vi "Configure Watchdog.vi"(5 "Dog stop notifier":refnum<notifier>, 7 "Period":i32, 8 "error in (no error)":errorcluster, 9 "Register":u16, 10 "Modbus Handle":refnum<class "Modbus Master.lvclass">, 11 "Watchdog in":refnum<class "Watchdog.lvclass">) -> (0 "error out":errorcluster, 3 "Watchdog out":refnum<class "Watchdog.lvclass">)   [LabVIEW 2015, in "Watchdog Actor.lvlib" / "Watchdog.lvclass"]
uses:
  Watchdog.lvclass
  <vilib>/Modbus/master/Modbus Master.lvclass
  Watchdog.lvclass/Watchdog.ctl
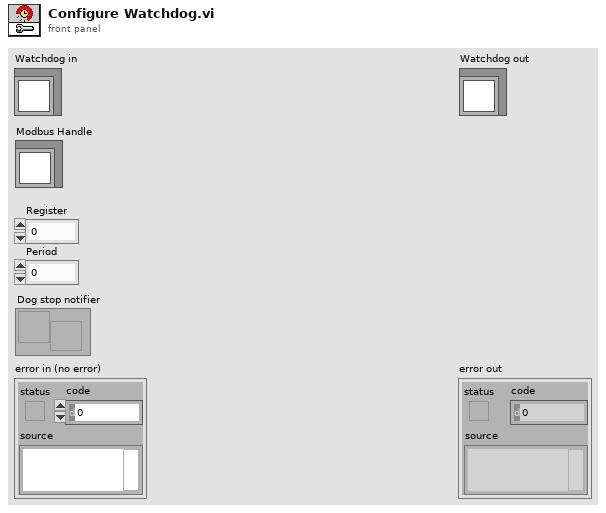
[diagram p1: front panel]
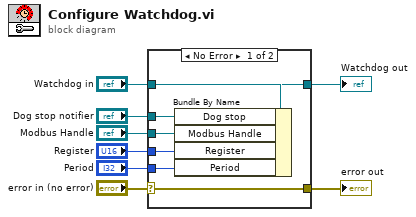
[diagram p0: block diagram]
diagram:
  n1 = case shown="No Error" "error in (no error)" {
    selector: "error in (no error)" -> [w14 w17]
    tunnel: [w14 w17] -> w7
    tunnel: [w13 w16] -> w5
    tunnel: "Watchdog in" -> [w15 w16]
    tunnel: "Register" -> [w12 _]
    tunnel: "Period" -> [w11 _]
    tunnel: "Modbus Handle" -> [w10 _]
    tunnel: "Dog stop notifier" -> [w9 _]
    frame No Error {
      n2 = Bundle By Name(cluster=w15, "Dog stop"=w9, "Modbus Handle"=w10, "Register"=w12, "Period"=w11) -> (w13:refnum<class "Watchdog.lvclass">)
    }
    frame Error {
    }
  }
  "error out" <- w7
  "Watchdog out" <- w5
